vi "Destination.vi"(0 "Root Destination In":path=path "", 1 "Root Folder Name":string) -> (2 "Root Destination Out":path)   [LabVIEW 2018, in "Scripts.lvlib"]
uses:
  Scripts.lvlib
  <vilib>/Field R&D Services/Labricator/Toolkit/Labricator.lvlib
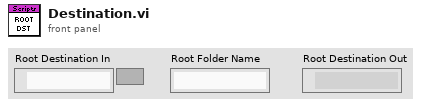
[diagram p1: front panel]
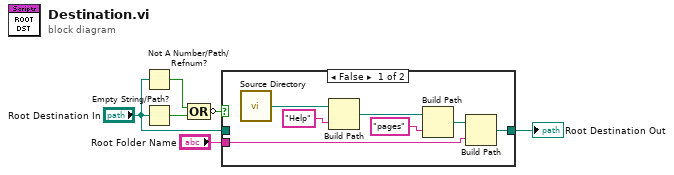
[diagram p0: block diagram]
diagram:
  n1 = Not A Number/Path/Refnum?(number/path/refnum="Root Destination In") -> (NaN/Path/Refnum?=w3:bool)
  n2 = Empty String/Path?(string/path="Root Destination In") -> (empty?=w2:bool)
  n3 = Compound Arithmetic op=OR(w3, w2) -> (invert w4:bool)
  n4 = case shown="False" w4 {
    tunnel: "Root Destination In" -> [_ w14]
    tunnel: [w8 w14] -> w6
    tunnel: "Root Folder Name" -> [w7 _]
    frame False {
      n5 = call <vilib>:"Source Directory.vi"() -> ("Source Directory"=w13:path)
      n6 = Build Path(base path=w13, name or relative path="Help") -> (appended path=w11:path)
      n7 = Build Path(base path=w11, name or relative path="pages") -> (appended path=w9:path)
      n8 = Build Path(base path=w9, name or relative path=w7) -> (appended path=w8:path)
    }
    frame True {
    }
  }
  "Root Destination Out" <- w6
